vi "Start Measurement.vi"(1 "Acquisition time":i32=1000 min=0 max=3600000 step=1, 2 "DeviceIndex":i32) -> (0 "DataValid":bool)   [LabVIEW 2011]
uses:
  MT Scan/SubVIs/hhlib.dll
panel:
  out "histolength":i32
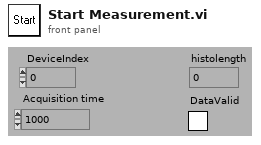
[diagram p1: front panel]
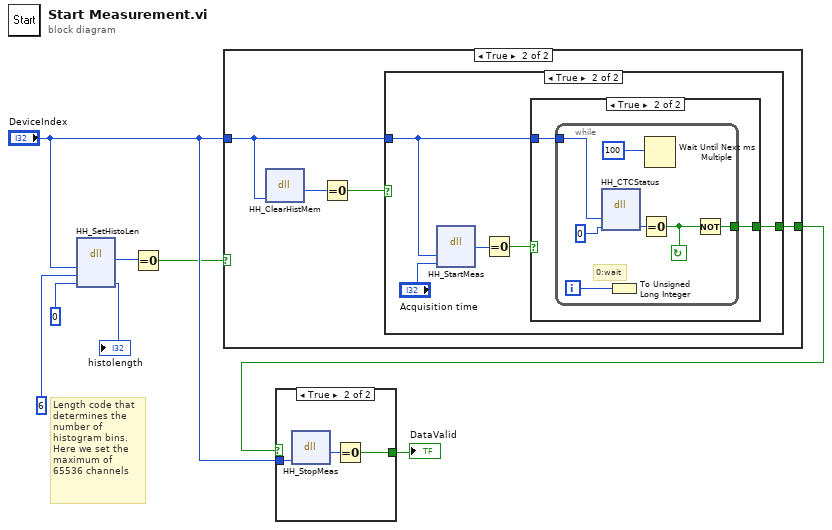
[diagram p0: block diagram]
diagram:
  # "Length code that \ndetermines the \nnumber of\nhistogram bins.\nHere we set the \nmaximum of\n65536 channels"
  n1 = dll-call lib="C:/Users/Core-FCS/Desktop/AbelFCS/MT Scan/SubVIs/hhlib.dll" fn="HH_SetHistoLen"("devidx"="DeviceIndex", "lencode"=6, "actuallen"=0) -> (w1:i32, "actuallen"=→"histolength":i32)  [unwired: 5 in, 2 out]
  n2 = Equal To 0?(x=w1) -> (x = 0?=w3:bool)
  n3 = case shown="True" w3 {
    selector: w3 -> [w9 _]
    tunnel: [w9 w13] -> w8
    tunnel: "DeviceIndex" -> [_ w11]
    frame False {
    }
    frame True {
      n4 = dll-call lib="C:/Users/Core-FCS/Desktop/AbelFCS/MT Scan/SubVIs/hhlib.dll" fn="HH_ClearHistMem"("devidx"=w11) -> (w12:i32)  [unwired: 4 in, 2 out]
      n5 = Equal To 0?(x=w12) -> (x = 0?=w10:bool)
      n6 = case shown="True" w10 {
        selector: w10 -> [w14 _]
        tunnel: [w14 w19] -> w13
        tunnel: w11 -> [_ w15]
        frame False {
        }
        frame True {
          n7 = dll-call lib="C:/Users/Core-FCS/Desktop/AbelFCS/MT Scan/SubVIs/hhlib.dll" fn="HH_StartMeas"("devidx"=w15, "tacq"="Acquisition time") -> (w17:i32)  [unwired: 5 in, 2 out]
          n8 = Equal To 0?(x=w17) -> (x = 0?=w16:bool)
          n9 = case shown="True" w16 {
            selector: w16 -> [w20 _]
            tunnel: [w20 w22] -> w19
            tunnel: w15 -> [_ w21]
            frame False {
            }
            frame True {
              n10 = while {
                tunnel: w21 -> [w24]
                tunnel: [w27] -> w22
                i -> [w26]
                stop <- w28 continue-if-true
                # "0:wait"
                n11 = dll-call lib="C:/Users/Core-FCS/Desktop/AbelFCS/MT Scan/SubVIs/hhlib.dll" fn="HH_CTCStatus"("devidx"=w24, "status"=0) -> ("status"=w23:i32)  [unwired: 5 in, 2 out]
                n12 = To Unsigned Long Integer(number=w26) -> ()  [unwired: 1 out]
                n13 = Equal To 0?(x=w23) -> (x = 0?=w28:bool)
                n14 = Wait Until Next ms Multiple(millisecond multiple=100) -> ()  [unwired: 1 out]
                n15 = Not(x=w28) -> (.not. x?=w27:bool)
              }
            }
          }
        }
      }
    }
  }
  n16 = case shown="True" w8 {
    selector: w8 -> [w30 _]
    tunnel: [w30 w33] -> w7
    tunnel: "DeviceIndex" -> [_ w32]
    frame False {
    }
    frame True {
      n17 = dll-call lib="C:/Users/Core-FCS/Desktop/AbelFCS/MT Scan/SubVIs/hhlib.dll" fn="HH_StopMeas"("devidx"=w32) -> (w31:i32)  [unwired: 4 in, 2 out]
      n18 = Equal To 0?(x=w31) -> (x = 0?=w33:bool)
    }
  }
  "DataValid" <- w7
